vi "Read Config From Device.vi"(8 "error in (no error)":errorcluster, 10 "Channel":string, 11 "Agilent DSO-X 3032A in":refnum<class "Agilent DSO-X 3032A.lvclass">) -> (0 "error out":errorcluster, 3 "Agilent DSO-X 3032A out":refnum<class "Agilent DSO-X 3032A.lvclass">)   [LabVIEW 2014, in "Agilent DSO-X 3032A.lvclass"]
uses:
  Agilent DSO-X 3032A.lvclass
  Agilent DSO-X 3032A.lvclass/Agilent DSO-X 3032A.ctl
  Channel Settings.ctl
  Framework/Interfaces/Observable Actor/Observable Actor.lvclass
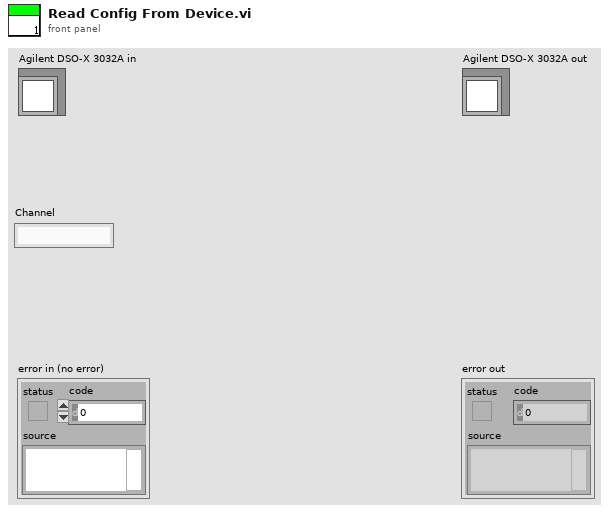
[diagram p1: front panel]
types:
  T1 = typedef "Agilent DSO-X 3032A.lvclass/Channel Settings.ctl" = cluster{"Dt":dbl, "#samples":i32, "t0":dbl}
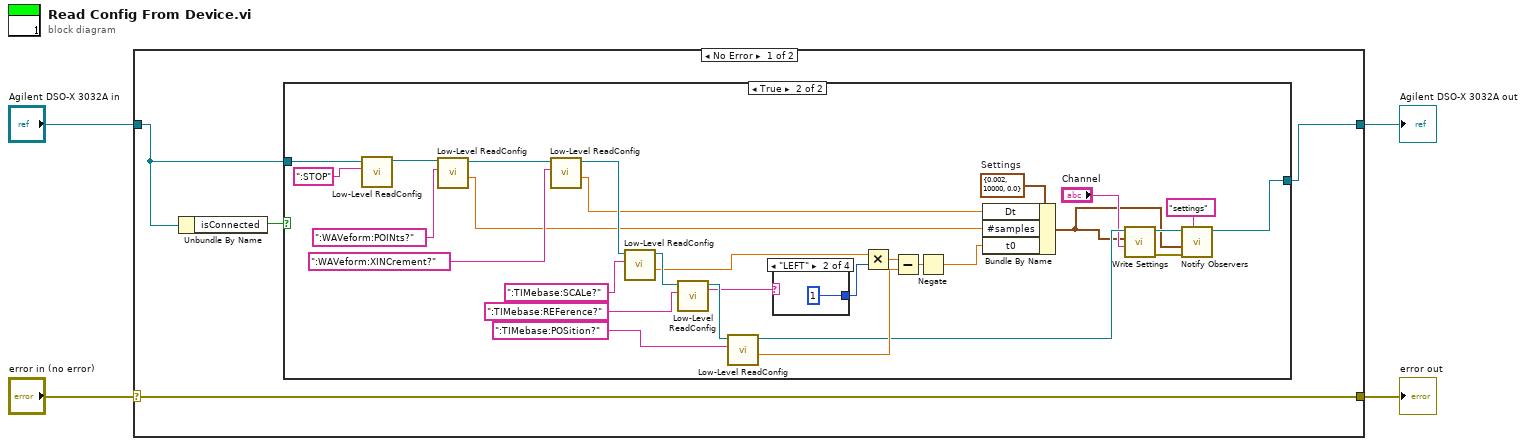
[diagram p0: block diagram]
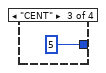
[diagram p4: hidden frame]
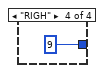
[diagram p5: hidden frame]
diagram:
  n1 = case shown="No Error" "error in (no error)" {
    selector: "error in (no error)" -> [w8 w43]
    tunnel: [w8 w43] -> w3
    tunnel: [w6 w42] -> w1
    tunnel: "Agilent DSO-X 3032A in" -> [w5 w42]
    frame No Error {
      n2 = Unbundle By Name(w5) -> ("isConnected"=w7:bool)
      n3 = case shown="True" w7 {
        tunnel: [w9 w19] -> w6
        tunnel: w5 -> [w9 w23]
        frame False {
        }
        frame True {
          w18 = T1 {"Dt"=0.002, "#samples"=10000, "t0"=0.0}  # Settings
          n4 = call "Low-Level ReadConfig.vi"("Command"=":STOP", "Agilent DSO-X 3032A in"=w23) -> ("Agilent DSO-X 3032A out"=w22:refnum<class "Agilent DSO-X 3032A.lvclass">)  [unwired: 6 in, 3 out]
          n5 = call "Low-Level ReadConfig.vi"("Command"=":WAVeform:POINts?", "Agilent DSO-X 3032A in"=w22) -> ("Data as DBL"=w16:dbl, "Agilent DSO-X 3032A out"=w24:refnum<class "Agilent DSO-X 3032A.lvclass">)  [unwired: 6 in, 2 out]
          n6 = call "Low-Level ReadConfig.vi"("Command"=":WAVeform:XINCrement?", "Agilent DSO-X 3032A in"=w24) -> ("Data as DBL"=w15:dbl, "Agilent DSO-X 3032A out"=w20:refnum<class "Agilent DSO-X 3032A.lvclass">)  [unwired: 6 in, 2 out]
          n7 = call "Low-Level ReadConfig.vi"("Command"=":TIMebase:SCALe?", "Agilent DSO-X 3032A in"=w20) -> ("Data as DBL"=w27:dbl, "Agilent DSO-X 3032A out"=w37:refnum<class "Agilent DSO-X 3032A.lvclass">)  [unwired: 6 in, 2 out]
          n8 = call "Low-Level ReadConfig.vi"("Command"=":TIMebase:REFerence?", "Agilent DSO-X 3032A in"=w37) -> ("Data"=w35:string, "Agilent DSO-X 3032A out"=w36:refnum<class "Agilent DSO-X 3032A.lvclass">)  [unwired: 6 in, 2 out]
          n9 = call "Low-Level ReadConfig.vi"("Command"=":TIMebase:POSition?", "Agilent DSO-X 3032A in"=w36) -> ("Data as DBL"=w26:dbl, "Agilent DSO-X 3032A out"=w14:refnum<class "Agilent DSO-X 3032A.lvclass">)  [unwired: 6 in, 2 out]
          n10 = case shown="\"LEFT\"" w35 {
            tunnel: [_ 1 5 9] -> w32
            frame Default {
            }
            frame "LEFT" {
            }
            frame "CENT" {
            }
            frame "RIGH" {
            }
          }
          n11 = Multiply(x=w27, y=w32) -> (x*y=w31:dbl)
          n12 = Subtract(x=w31, y=w26) -> (x-y=w29:dbl)
          n13 = Negate(x=w29) -> (-x=w17:dbl)
          n14 = Bundle By Name(cluster=w18, "Dt"=w15, "#samples"=w16, "t0"=w17) -> (w10:T1)
          n15 = call "Write Settings.vi"("Channel"="Channel", "Settings"=w10, "Agilent DSO-X 3032A in"=w14) -> ("error out"=w11:errorcluster, "Agilent DSO-X 3032A out"=w13:refnum<class "Agilent DSO-X 3032A.lvclass">)  [unwired: 7 in]
          n16 = call "Notify Observers.vi"("name"="settings", "error in (no error)"=w11, "value"=w10, "Observable Actor in"=w13) -> ("Observable Actor out"=w19:refnum<class "Agilent DSO-X 3032A.lvclass">)  [unwired: 6 in, 1 out]
        }
      }
    }
    frame Error {
    }
  }
  "error out" <- w3
  "Agilent DSO-X 3032A out" <- w1
